vi "Get Base Command.vi"(8 "error in (no error)":errorcluster, 11 "User Defined Read in":refnum<class "User Defined Read.lvclass">) -> (0 "error out":errorcluster, 2 "Base Command":string, 3 "User Defined Read out":refnum<class "User Defined Read.lvclass">)   [LabVIEW 2023, in "HAF.lvlib" / "User Defined Read.lvclass"]
doc: "Returns the base command whch is used to build up the overall command string – parameters will be added to this as necessary.  The framework will add the line terminator \\n.\n\nSubclasses MUST override this member and must not add a line terminator on the end of the command; on this class an error is returned."
uses:
  User Defined Read.lvclass
  User Defined Read.lvclass/User Defined Read.ctl
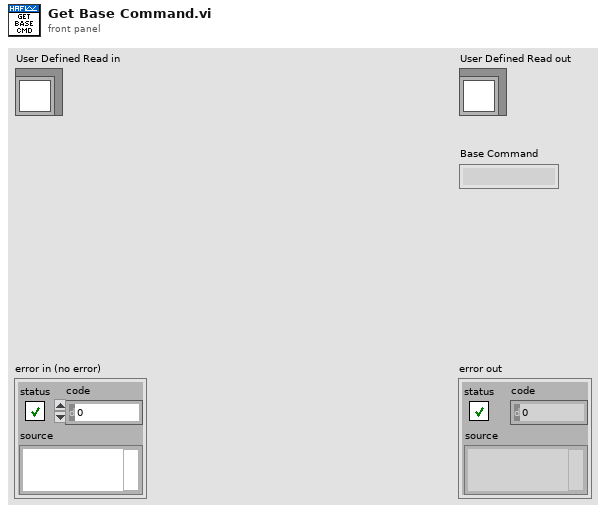
[diagram p1: front panel]
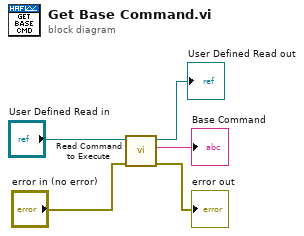
[diagram p0: block diagram]
diagram:
  n1 = call-dynamic "Read Command to Execute.vi"("error in (no error)"="error in (no error)", "User Defined Read in"="User Defined Read in") -> ("error out"=→"error out":errorcluster, "Command to Execute"=→"Base Command":string, "User Defined Read out"=→"User Defined Read out":refnum<class "User Defined Read.lvclass">)  [unwired: 7 in]
